vi "XML_FF_readHeader.vi"(8 "error in (no error)":errorcluster, 11 "DOM document in":refnum<k20>) -> (0 "error out":errorcluster, 2 "FF_Header out":T1, 3 "DOM document out":refnum<k20>)   [LabVIEW 2016, in "XML_EEG_Features.lvlib"]
doc: "Прочитать заголовок XML файла, содержащего рассчитанные значения спектра сигнала ЭЭГ"
uses:
  XML_EEG_Features.lvlib
  XML_FF_Header.ctl
  <vilib>/xml/NI_XML.lvlib
panel:
  # "This VI is a part of BCI Design library, http://www.ru-bci.org \nCopyright © 2020, Sotnikov Peter, All rights reserved. License: GNU GPLv3"
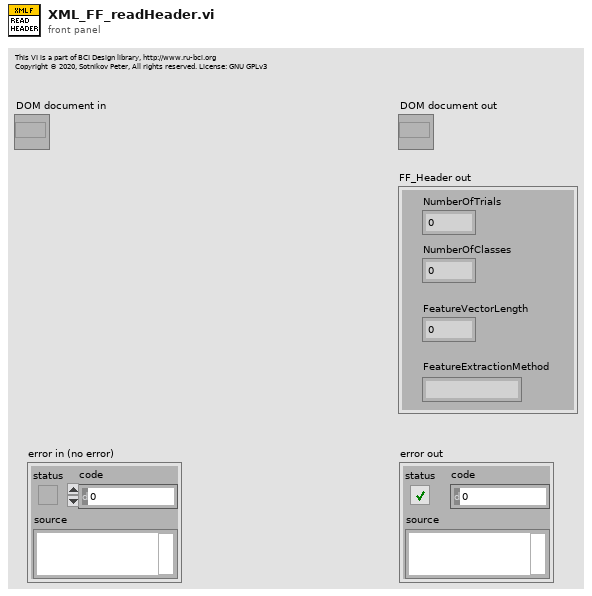
[diagram p1: front panel]
types:
  T1 = typedef "XML_EEG_Features.lvlib/XML_FF_Header.ctl" = cluster{"NumberOfTrials":i32, "NumberOfClasses":i32, "FeatureVectorLength":i32, "FeatureExtractionMethod":string}
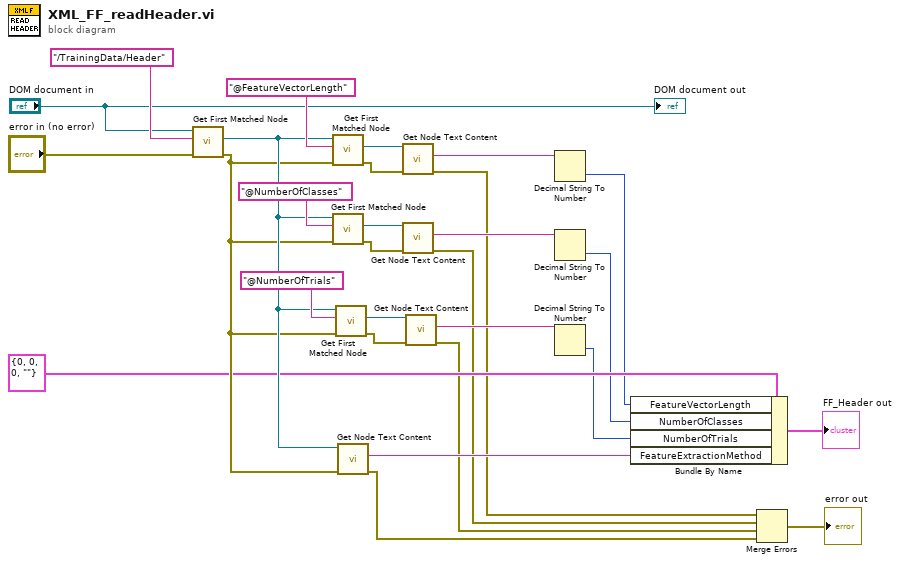
[diagram p0: block diagram]
diagram:
  n1 = call <vilib>:"Get First Matched Node.vi"("error in (no error)"="error in (no error)", "XPath expression"="/TrainingData/Header", "node in"="DOM document in") -> ("error out"=w13:errorcluster, "node result"=w14:refnum<k20>)  [unwired: 6 in, 1 out]
  n2 = call <vilib>:"Get First Matched Node.vi"("error in (no error)"=w13, "XPath expression"="@FeatureVectorLength", "node in"=w14) -> ("error out"=w25:errorcluster, "node result"=w26:refnum<k20>)  [unwired: 6 in, 1 out]
  n3 = call <vilib>:"Get First Matched Node.vi"("error in (no error)"=w13, "XPath expression"="@NumberOfClasses", "node in"=w14) -> ("error out"=w22:errorcluster, "node result"=w23:refnum<k20>)  [unwired: 6 in, 1 out]
  n4 = call <vilib>:"Get First Matched Node.vi"("error in (no error)"=w13, "XPath expression"="@NumberOfTrials", "node in"=w14) -> ("error out"=w20:errorcluster, "node result"=w21:refnum<k20>)  [unwired: 6 in, 1 out]
  n5 = call <vilib>:"Get Node Text Content.vi"("error in (no error)"=w13, "node in"=w14) -> ("error out"=w4:errorcluster, "node text"=w8:string)  [unwired: 7 in, 1 out]
  n6 = call <vilib>:"Get Node Text Content.vi"("error in (no error)"=w25, "node in"=w26) -> ("error out"=w7:errorcluster, "node text"=w24:string)  [unwired: 7 in, 1 out]
  n7 = call <vilib>:"Get Node Text Content.vi"("error in (no error)"=w22, "node in"=w23) -> ("error out"=w6:errorcluster, "node text"=w16:string)  [unwired: 7 in, 1 out]
  n8 = call <vilib>:"Get Node Text Content.vi"("error in (no error)"=w20, "node in"=w21) -> ("error out"=w5:errorcluster, "node text"=w15:string)  [unwired: 7 in, 1 out]
  n9 = Decimal String To Number(string=w24) -> (number=w11:i32)  [unwired: 2 in, 1 out]
  n10 = Decimal String To Number(string=w16) -> (number=w10:i32)  [unwired: 2 in, 1 out]
  n11 = Decimal String To Number(string=w15) -> (number=w9:i32)  [unwired: 2 in, 1 out]
  n12 = Bundle By Name(cluster=T1 {"NumberOfTrials"=0, "NumberOfClasses"=0, "FeatureVectorLength"=0, "FeatureExtractionMethod"=""} ("XML_FF_Header"), "FeatureVectorLength"=w11, "NumberOfClasses"=w10, "NumberOfTrials"=w9, "FeatureExtractionMethod"=w8) -> (→"FF_Header out":T1)
  n13 = Merge Errors(w7, w6, w5, w4) -> (→"error out":errorcluster)
  "DOM document out" <- "DOM document in"
